vi "Test - Indicators.vi"(8 "error in (no error)":errorcluster) -> (0 "error out":errorcluster)   [LabVIEW 2020]
doc: "Dummy test."
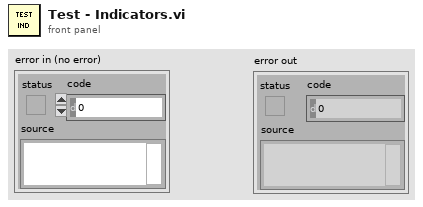
[diagram p1: front panel]
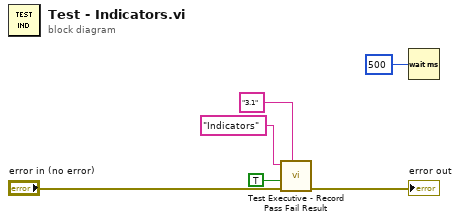
[diagram p0: block diagram]
diagram:
  n1 = call "Test Executive - Record Pass Fail Result.vi"("Test Ref"="3.1", "error in (no error)"="error in (no error)", "Pass"=TRUE, "Test Name"="Indicators") -> ("error out"=→"error out":errorcluster)  [unwired: 7 in]
  n2 = Wait (ms)(milliseconds to wait=u32 500) -> ()  [unwired: 1 out]
